vi "Dummy map producer.vi"   [LabVIEW 2012]
uses:
  <vilib>/Platform/TimedLoop/XDataNode/timing_clust.ctl
  <vilib>/Platform/TimedLoop/XDataNode/nitl_modes.ctl
  <vilib>/Platform/TimedLoop/XDataNode/wakeup.ctl
  <vilib>/Platform/TimedLoop/XDataNode/XDataNode.xnode
  <vilib>/robotics/Navigation/shared/WorldMap/OccupancyGridWorldMap/NI_Robotics_OccupancyGridWorldMap.lvclass
  <vilib>/Platform/TimedLoop/XDataNode/XDNodeRunTimeDep.lvlib
types:
  T1 = typedef "XDNodeRunTimeDep.lvlib/timing_clust.ctl" = cluster{"Expected End [f-1]":u64, "Actual End [f-1]":u64, "Finished Late? [f-1]":bool, "Expected End [i-1]":u64, "Actual End [i-1]":u64, "Finished Late? [i-1]":bool, "Expected Start [i]":u64, "Actual Start [i]":u64, "Expected Start [f]":u64, "Actual Start [f]":u64, "Source Name":string, "Structure Name":string, "Period":i64, "Deadline":i64, "Offset":i64, "Start":i64, "Priority":i32, "Timeout":i32, "Mode":T2, "Wakeup Reason":T3, "Error":errorcluster, "Source Type":string, "Secondary Source Type":string, "Global End Time":u64, "Global Start Time":u64, "Frame Duration":u64, "Iteration Duration":u64, "Assigned CPU":i32, "I/O Scan Engine Mode":u32}
  T2 = typedef "XDNodeRunTimeDep.lvlib/nitl_modes.ctl" = enum32{"No Change", "Process missed periods, maintain original phase", "Discard missed periods, maintain original phase", "Process missed periods, ignore original phase", "Discard missed periods, ignore original phase"}
  T3 = typedef "XDNodeRunTimeDep.lvlib/wakeup.ctl" = enum32{"Normal", "Aborted", "Asynchronous wakeup", "Timing source error", "Timed loop error", "Timeout"}
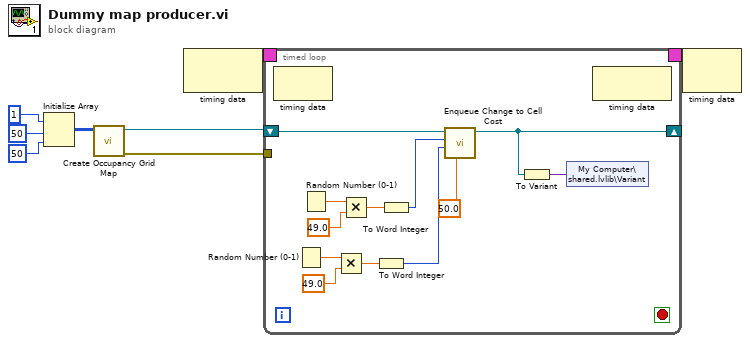
[diagram p0: block diagram]
diagram:
  n1 = Initialize Array(1, 50, 50) -> (w5:i32[][])
  n2 = call <vilib>:"Create Occupancy Grid Map.vi"("occupancy grid"=w5) -> ("error out"=w1:errorcluster, "map reference out"=w2:refnum<data-value>)  [unwired: 9 in]
  n3 = node-c288() -> (w4:T1)  [unwired: 1 in]
  n4 = timed-loop {
    timing: w4 -> [_]
    timing-out: [_] -> w3
    tunnel: w1 -> [_]
    shift-right: [w10] -> _
    shift-left: w2 -> [w20]
    stop <- _ stop-if-true
    n5 = node-c288() -> ()  [unwired: 1 in, 1 out]
    n6 = Random Number (0-1)() -> (number: 0 to 1=w13:dbl)
    n7 = Random Number (0-1)() -> (number: 0 to 1=w19:dbl)
    n8 = Multiply(x=w13, y=49.0) -> (x*y=w15:dbl)
    n9 = Multiply(x=w19, y=49.0) -> (x*y=w17:dbl)
    n10 = To Word Integer(number=w15) -> (16bit integer=w12:i16)
    n11 = To Word Integer(number=w17) -> (16bit integer=w16:i16)
    n12 = call <vilib>:"Enqueue Change to Cell Cost.vi"("cost"=50.0, "y"=w12, "x"=w16, "map reference in"=w20) -> ("map reference out"=w10:refnum<data-value>)  [unwired: 6 in, 1 out]
    n13 = To Variant(anything=w10) -> (Variant=w9:variant)
    n14 = shared-variable "My Computer\\shared.lvlib\\Variant"(w9) -> ()  [unwired: 1 in, 1 out]
    n15 = node-c288() -> ()  [unwired: 1 in, 1 out]
  }
  n16 = node-c288(w3) -> ()  [unwired: 1 out]
